vi "Card_output_host.vi"() -> ()   [LabVIEW 2015]
uses:
  <vilib>/userdefined/High Color/nirio_resource_hc.ctl
  <vilib>/FPGAPlugInAG/PXIe-7962R/niLvFpga_Open_PXIe-7962R.vi
  <vilib>/rvi/interface/common/dynamic/niFpgaDynamicAddResources.vi
  <vilib>/LabVIEW Targets/FPGA/FlexRIO/CustomFPGAMethods/79XXR_Method_IOModuleStatusImpl.vi
  <vilib>/Utility/error.llb/Error Cluster From Error Code.vi
  <vilib>/rvi/errors/niLvFpgaAdjustHostInterfaceError.vi
  <vilib>/rvi/interface/common/niFpgaWaitOnOcc.vi
  <instrlib>/_niInstr/Streaming/v1/Host/Public/Start Finite Stream.vi
  <instrlib>/niSync/niSync.llb/niSync Initialize (IVI).vi
  <instrlib>/_niInstr/Streaming/v1/Host/Public/Wait for Stream.vi
  <vilib>/FPGAPlugInAG/Dynamic/niLvFpga_Close_Dynamic.vi
  <vilib>/rvi/interface/nirviOpenFPGA/nirviOpenFPGA.xnode
  FPGA Bitfiles/MochiFPGAControl_FPGATarget_pxie7962fpga_vH47uBXjtQs.lvbitx
  <vilib>/rvi/interface/nirviMethod/nirviMethod.xnode
  <vilib>/rvi/interface/nirviReadWriteControl/nirviReadWriteControl.xnode
  <vilib>/rvi/interface/nirviCloseFPGA/nirviCloseFPGA.xnode
  <instrlib>/_niInstr/Streaming/v1/Host/niInstr Streaming v1 Host.lvlib
  <vilib>/rvi/errors/niLvFpgaMergeErrorWithErrorCode.vi
  <vilib>/rvi/interface/Simulation/niFpgaSimulationCallBeginRW.vi
  NiFpgaLv.dll
  <vilib>/FPGAPlugInAG/Dynamic/niLvFpga_StartFifo_Dynamic.vi
  <vilib>/FPGAPlugInAG/Dynamic/niLvFpga_ReadFifo_Dynamic.vi
  <vilib>/FPGAPlugInAG/Dynamic/niLvFpga_ConfigureFifo_Dynamic.vi
  <vilib>/FPGAPlugInAG/Dynamic/niLvFpga_StopFifo_Dynamic.vi
panel:
  out "subarray":i16[](array[numeric])
  out "size(s) 2":i32[](array[numeric])
  out "size(s)":i32[](array[numeric])
  in  "Trigger destination terminal":string(combo)="PXI_Trig0"
  in  "FPGA":T1 caption="RIO Device"
  out "Bits out DRAM":u64
  out "Writes to DRAM":u64
  in  "?":enum32{"All AI individual", "All AI", "Al 0"}(tab)
  out "AI 31":i32[](graph)
  out "AI 30":i32[](graph)
  out "AI 29":i32[](graph)
  out "AI 28":i32[](graph)
  out "AI 27":i32[](graph)
  out "AI 26":i32[](graph)
  out "AI 25":i32[](graph)
  out "AI 24":i32[](graph)
  out "AI 23":i32[](graph)
  out "AI 22":i32[](graph)
  out "AI 21":i32[](graph)
  out "AI 20":i32[](graph)
  out "AI 19":i32[](graph)
  out "AI 18":i32[](graph)
  out "AI 17":i32[](graph)
  out "AI 16":i32[](graph)
  out "AI 15":i32[](graph)
  out "AI 14":i32[](graph)
  out "AI 13":i32[](graph)
  out "AI 12":i32[](graph)
  out "AI 11":i32[](graph)
  out "AI 10":i32[](graph)
  out "AI 9":i32[](graph)
  out "AI 8":i32[](graph)
  out "AI 7":i32[](graph)
  out "AI 6":i32[](graph)
  out "AI 5":i32[](graph)
  out "AI 4":i32[](graph)
  out "AI 3":i32[](graph)
  out "AI 2":i32[](graph)
  out "AI 1":i32[](graph)
  out "AI 0":i32[](graph)
  out "All AI":waveform(dbl)[](graph)
  out "just AI 1":waveform(dbl)(graph)
  in  "Debug":bool
  out "Bits out DMA":u64
  out "Bits aquired":u64
  out "Writes to DMA":u64
  out "Samples Aquired":u64
  out "Voltage":dbl[][](array[numeric])
  out "Counts":i16[][](array[numeric])
  out "error out":errorcluster
  out "samples transferred":u64
  out "Raw DMA readout":u64[](array[numeric])
  in  "num samples":u64=40000
  in  "Go":bool
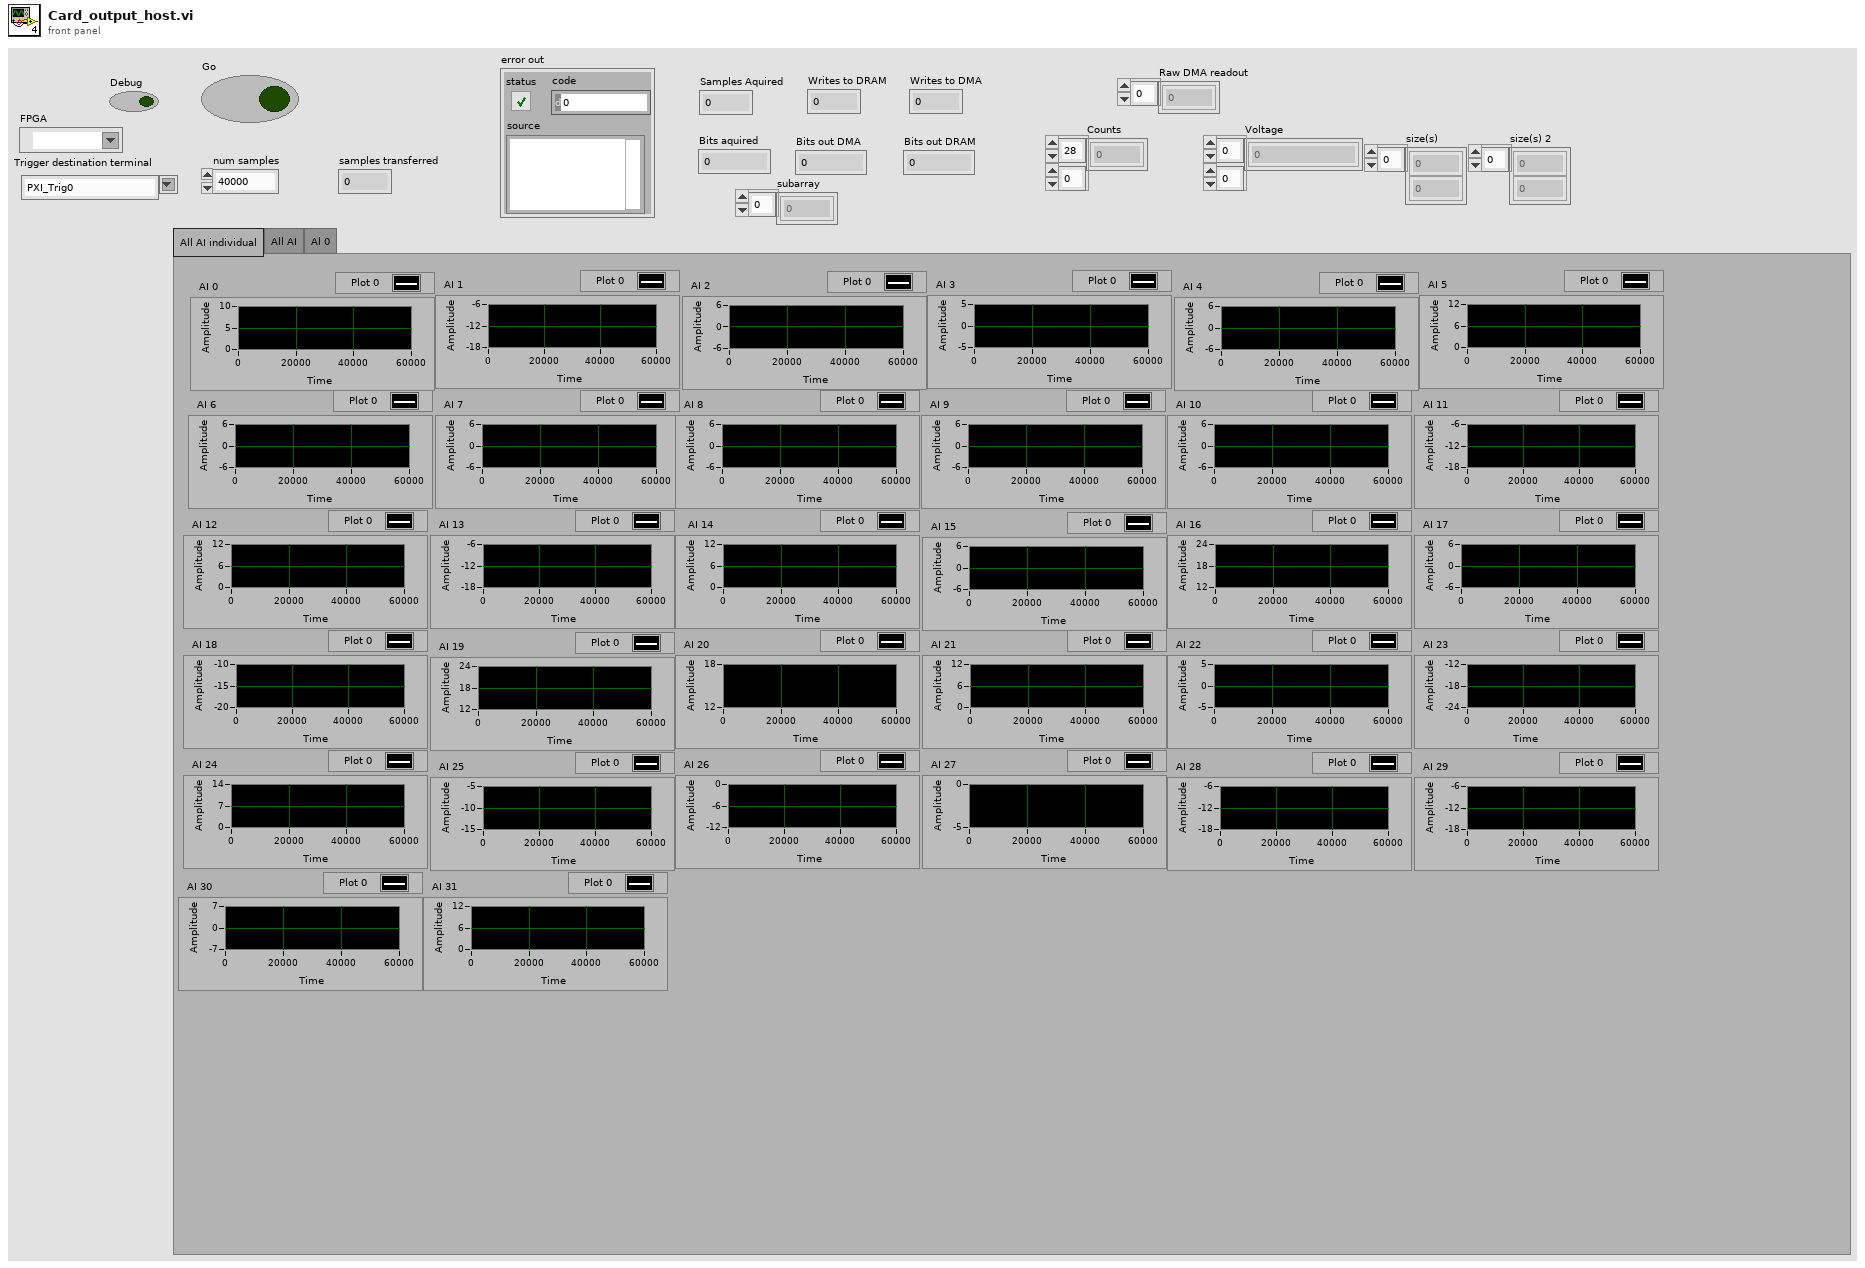
[diagram p1: front panel]
types:
  T1 = typedef "nirio_resource_hc.ctl" = tag
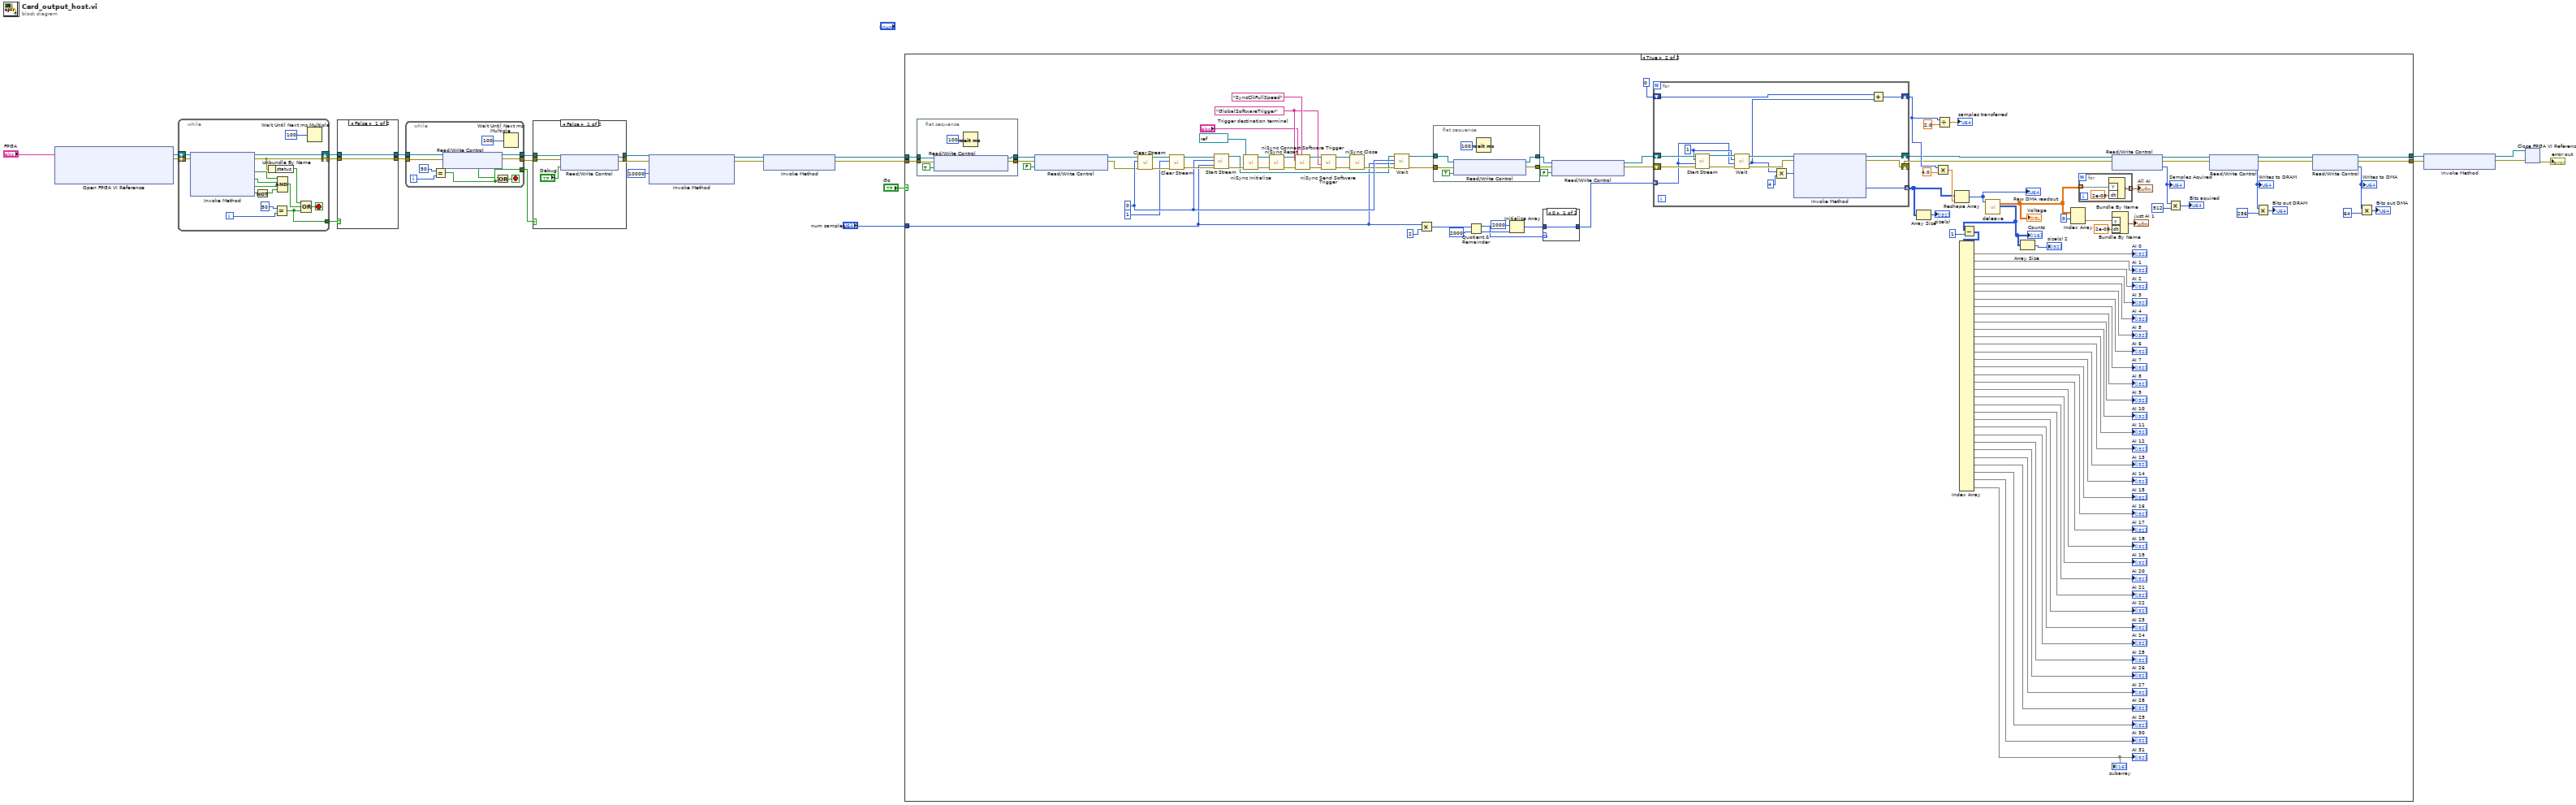
[diagram p0: block diagram]
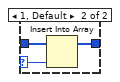
[diagram p3: hidden frame]
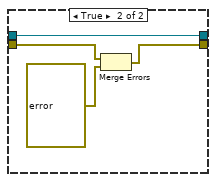
[diagram p4: hidden frame]
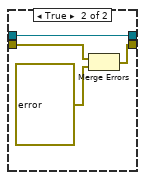
[diagram p5: hidden frame]
diagram:
  n1 = xnode "Open FPGA VI Reference"("resource name"="FPGA") -> ("FPGA VI Reference Out"=w10:refnum<k20>, "error out"=w11:errorcluster)  [unwired: 1 in]
  n2 = while {
    shift-right: [w32] -> w18
    shift-left: w11 -> [w40]
    shift-right: [w39] -> w16
    shift-left: w10 -> [w41]
    tunnel: [w28] -> w17
    i -> [w34]
    stop <- w29 stop-if-true
    n3 = xnode "Invoke Method"("FPGA VI Reference In"=w41, "error in"=w40) -> ("FPGA VI Reference Out"=w39:refnum<k20>, "error out"=w32:errorcluster, "IO Module Present?"=w38:bool, "Power Enabled?"=w37:bool, "IO Enabled?"=w36:bool, "IO Module Mismatch?"=w27:bool)
    n4 = Not(x=w27) -> (.not. x?=w26:bool)
    n5 = Unbundle By Name(w32) -> ("status"=w31:bool)
    n6 = Equal?(x=50, y=w34) -> (x = y?=w28:bool)
    n7 = Compound Arithmetic op=AND(w38, w37, w36, w26) -> (w30:bool)
    n8 = Compound Arithmetic op=OR(w31, w30, w28) -> (w29:bool)
    n9 = Wait Until Next ms Multiple(millisecond multiple=u32 100) -> ()  [unwired: 1 out]
  }
  n10 = case shown="False" w17 {
    tunnel: w18 -> [w42 w46]
    tunnel: [w42 w45] -> w14
    tunnel: w16 -> [w43 w44]
    tunnel: [w43 w44] -> w15
    frame False {
    }
    frame True {
      n11 = Merge Errors(w46, errorcluster {"status"=TRUE, "code"=-1, "source"="The IO Module was not present, powered, or the IO were not enabled.  Verify the NI 5752 is securly connected and try again."} ("error in")) -> (w45:errorcluster)
    }
  }
  n12 = while {
    tunnel: w15 -> [w52]
    tunnel: [w49] -> w8
    tunnel: [w50] -> w7
    tunnel: [w53] -> w9
    tunnel: w14 -> [w51]
    i -> [w56]
    stop <- w54 stop-if-true
    n13 = Equal?(x=50, y=w56) -> (x = y?=w53:bool)
    n14 = xnode "Read/Write Control"("FPGA VI Reference In"=w52, "error in"=w51) -> ("FPGA VI Reference Out"=w49:refnum<k20>, "error out"=w50:errorcluster, "IO Module Init Done"=w48:bool)
    n15 = Or(x=w48, y=w53) -> (x .or. y?=w54:bool)
    n16 = Wait Until Next ms Multiple(millisecond multiple=u32 100) -> ()  [unwired: 1 out]
  }
  n17 = case shown="False" w9 {
    tunnel: w7 -> [w59 w65]
    tunnel: [w58 w64] -> w12
    tunnel: w8 -> [w62 w63]
    tunnel: [w61 w63] -> w13
    frame False {
      n18 = xnode "Read/Write Control"("FPGA VI Reference In"=w62, "error in"=w59, "Output Debug Data"="Debug") -> ("FPGA VI Reference Out"=w61:refnum<k20>, "error out"=w58:errorcluster)
    }
    frame True {
      n19 = Merge Errors(w65, errorcluster {"status"=TRUE, "code"=-1, "source"="The IO Module CLIP was not ready. If you are using any external clocks, make sure they are connected and within the supported specifications."} ("error in")) -> (w64:errorcluster)
    }
  }
  n20 = xnode "Invoke Method"("FPGA VI Reference In"=w13, "error in"=w12, "Requested Depth"=u32 10000) -> ("FPGA VI Reference Out"=w24:refnum<k20>, "error out"=w23:errorcluster)  [unwired: 1 out]
  n21 = xnode "Invoke Method"("FPGA VI Reference In"=w24, "error in"=w23) -> ("FPGA VI Reference Out"=w22:refnum<k20>, "error out"=w21:errorcluster)
  n22 = case shown="True" "Go" {
    tunnel: w22 -> [w68 w161]
    tunnel: "num samples" -> [_ w70]
    tunnel: [w68 w131] -> w4
    tunnel: w21 -> [w67 w130]
    tunnel: [w67 w129] -> w3
    frame False {
      (unwired) errorcluster {"status"=FALSE, "code"=0, "source"=""} ("error out")
    }
    frame True {
      w120 = "GlobalSoftwareTrigger" ("source terminal")
      w176 = 0 ("stream index")
      n23 = flat-sequence {
        tunnel: [w213] -> w164
        tunnel: w161 -> [w212]
        tunnel: [w211] -> w160
        tunnel: w130 -> [w210]
        frame #0 {
          n24 = xnode "Read/Write Control"("FPGA VI Reference In"=w212, "error in"=w210, "Reset DRAM write address"=TRUE) -> ("FPGA VI Reference Out"=w211:refnum<k20>, "error out"=w213:errorcluster)
          n25 = Wait (ms)(milliseconds to wait=u32 100) -> ()  [unwired: 1 out]
        }
      }
      n26 = xnode "Read/Write Control"("FPGA VI Reference In"=w160, "error in"=w164, "Reset DRAM write address"=FALSE) -> ("FPGA VI Reference Out"=w140:refnum<k20>, "error out"=w145:errorcluster)
      n27 = call <instrlib>:"Clear Stream.vi"("error in (no error)"=w145, "stream index"=w176, "refnum in"=w140) -> ("error out"=w179:errorcluster, "refnum out"=w180:refnum<k20>)  [unwired: 7 in]
      n28 = call <instrlib>:"Clear Stream.vi"("error in (no error)"=w179, "stream index"=1, "refnum in"=w180) -> ("error out"=w177:errorcluster, "refnum out"=w178:refnum<k20>)  [unwired: 7 in]
      n29 = call-poly <instrlib>:"Start Stream.vi"("error in (no error)"=w177, "num samples"=w70, "stream index"=w176, "refnum in"=w178) -> ("error out"=w126:errorcluster, "refnum out"=w119:refnum<k20>)  [unwired: 6 in]
      n30 = call-poly <instrlib>:"niSync Initialize.vi"("error in (no error)"=w126, "resource name"=refnum<k15> "Sync1") -> ("error out"=w77:errorcluster, "instrument handle out"=w78:refnum<k15>)  [unwired: 8 in]
      n31 = call <instrlib>:"niSync Reset.vi"("error in (no error)"=w77, "instrument handle"=w78) -> ("error out"=w75:errorcluster, "instrument handle out"=w76:refnum<k15>)  [unwired: 8 in]
      n32 = call <instrlib>:"niSync Connect Software Trigger.vi"("synchronization clock"="SyncClkFullSpeed", "error in (no error)"=w75, "destination terminal"="Trigger destination terminal", "source terminal"=w120, "instrument handle"=w76) -> ("error out"=w128:errorcluster, "instrument handle out"=w127:refnum<k15>)  [unwired: 5 in]
      n33 = call <instrlib>:"niSync Send Software Trigger.vi"("error in (no error)"=w128, "source terminal"=w120, "instrument handle"=w127) -> ("error out"=w124:errorcluster, "instrument handle out"=w125:refnum<k15>)  [unwired: 7 in]
      n34 = call <instrlib>:"niSync Close.vi"("error in (no error)"=w124, "instrument handle"=w125) -> ("error out"=w123:errorcluster)  [unwired: 9 in]
      n35 = call-poly <instrlib>:"Wait.vi"("error in (no error)"=w123, "wait for samples transferred"=w70, "stream index"=w176, "refnum in"=w119) -> ("error out"=w69:errorcluster, "refnum out"=w159:refnum<k20>)  [unwired: 4 in, 2 out]
      n36 = Multiply(x=w70, y=u64 2) -> (x*y=w151:u64)
      n37 = flat-sequence {
        tunnel: [w207] -> w162
        tunnel: w159 -> [w206]
        tunnel: [w205] -> w158
        tunnel: w69 -> [w204]
        frame #0 {
          n38 = xnode "Read/Write Control"("FPGA VI Reference In"=w206, "error in"=w204, "Reset DRAM read address"=TRUE ("Reset DRAM write address")) -> ("FPGA VI Reference Out"=w205:refnum<k20>, "error out"=w207:errorcluster)
          n39 = Wait (ms)(milliseconds to wait=u32 100) -> ()  [unwired: 1 out]
        }
      }
      n40 = Quotient & Remainder(x=w151, y=u64 2000) -> (x-y*floor(x/y)=w141:u64, floor(x/y)=w149:u64)
      n41 = Initialize Array(u64 2000 ("element"), w149) -> (w147:u64[])
      n42 = case shown="0" w141 {
        selector: w141 -> [_ w185]
        tunnel: w147 -> [w184 w187]
        tunnel: [w184 w186] -> w146
        frame 0 {
        }
        frame 1, Default {
          n43 = Insert Into Array(array=w187, new element=w185) -> (w186:u64[])  [unwired: 1 in]
        }
      }
      n44 = xnode "Read/Write Control"("FPGA VI Reference In"=w158, "error in"=w162, "Reset DRAM read address"=FALSE ("Reset DRAM write address")) -> ("FPGA VI Reference Out"=w152:refnum<k20>, "error out"=w153:errorcluster)
      n45 = for {
        shift-right: [w190] -> w144
        shift-left: w152 -> [w200]
        shift-right: [w189] -> w139
        shift-left: w153 -> [w199]
        shift-right: [w203] -> w155
        shift-left: u64 0 -> [w197]
        tunnel: w146 -> [w188] mode=indexing
        tunnel: [w191] -> w81 mode=indexing
        w198 = 1 ("stream index")
        n46 = call-poly <instrlib>:"Start Stream.vi"("error in (no error)"=w199, "num samples"=w188, "stream index"=w198, "refnum in"=w200) -> ("error out"=w201:errorcluster, "refnum out"=w202:refnum<k20>)  [unwired: 6 in]
        n47 = call-poly <instrlib>:"Wait.vi"("error in (no error)"=w201, "wait for samples transferred"=w188, "stream index"=w198, "refnum in"=w202) -> ("error out"=w195:errorcluster, "samples transferred"=w193:u64, "refnum out"=w196:refnum<k20>)  [unwired: 4 in, 1 out]
        n48 = Multiply(x=w193, y=u64 4) -> (x*y=w194:u64)
        n49 = xnode "Invoke Method"("FPGA VI Reference In"=w196, "error in"=w195, "Number of Elements"=w194) -> ("FPGA VI Reference Out"=w190:refnum<k20>, "error out"=w189:errorcluster, "Data"=w191:u64[])  [unwired: 1 in, 1 out]
        n50 = Add(x=w197, y=w193) -> (x+y=w203:u64)
      }
      n51 = Array Size(array=w81) -> (size(s)=→"size(s)":i32[])
      n52 = Multiply(x=w155, y=4.0) -> (x*y=w143:dbl)
      n53 = Divide(x=w155, y=2.0) -> (x/y=→"samples transferred":dbl)
      n54 = Reshape Array(w81, w143) -> (w142:u64[])
      "Raw DMA readout" <- w142
      n55 = call "deleave.vi"("Data"=w142) -> ("Counts"=w73:i16[][], "Voltage"=w74:dbl[][])  [unwired: 9 in]
      "Voltage" <- w74
      "Counts" <- w73
      n56 = Subtract(x=w73, y=1) -> (x-y=w71:i32[][])
      n57 = Index Array(array=w71) -> (element #1=→"AI 0":i32[], element #2=→"AI 1":i32[], element #3=→"AI 2":i32[], element #4=→"AI 3":i32[], element #5=→"AI 4":i32[], element #6=→"AI 5":i32[], element #7=→"AI 6":i32[], element #8=→"AI 7":i32[], element #9=→"AI 8":i32[], element #10=→"AI 9":i32[], element #11=→"AI 10":i32[], element #12=→"AI 11":i32[], element #13=→"AI 12":i32[], element #14=→"AI 13":i32[], element #15=→"AI 14":i32[], element #16=→"AI 15":i32[], element #17=→"AI 16":i32[], element #18=→"AI 17":i32[], element #19=→"AI 18":i32[], element #20=→"AI 19":i32[], element #21=→"AI 20":i32[], element #22=→"AI 21":i32[], element #23=→"AI 22":i32[], element #24=→"AI 23":i32[], element #25=→"AI 24":i32[], element #26=→"AI 25":i32[], element #27=→"AI 26":i32[], element #28=→"AI 27":i32[], element #29=→"AI 28":i32[], element #30=→"AI 29":i32[], element #31=→"AI 30":i32[], element #32=→"AI 31" →"subarray":i32[])  [unwired: 64 in]
      n58 = Array Size(array=w73) -> (size(s)=→"size(s) 2":i32[])
      n59 = Index Array(array=w74, index (row)=0) -> (element=w117:dbl[])  [unwired: 1 in]
      n60 = for {
        tunnel: [w183] -> w115 mode=indexing
        tunnel: w74 -> [w182] mode=indexing
        n61 = Bundle By Name("Y"=w182, "dt"=2e-08) -> (w183:waveform(dbl))  [unwired: 1 in]
      }
      "All AI" <- w115
      n62 = xnode "Read/Write Control"("FPGA VI Reference In"=w144, "error in"=w139) -> ("FPGA VI Reference Out"=w135:refnum<k20>, "error out"=w134:errorcluster, "Samples Aquired"=w172:u64)
      "Samples Aquired" <- w172
      n63 = Bundle By Name("Y"=w117, "dt"=2e-08) -> (→"just AI 1":waveform(dbl))  [unwired: 1 in]
      n64 = Multiply(x=w172, y=u64 512) -> (x*y=→"Bits aquired":u64)
      n65 = xnode "Read/Write Control"("FPGA VI Reference In"=w135, "error in"=w134) -> ("FPGA VI Reference Out"=w133:refnum<k20>, "error out"=w132:errorcluster, "Writes to DRAM"=w137:u64)
      "Writes to DRAM" <- w137
      n66 = Multiply(x=w137, y=u64 256) -> (x*y=→"Bits out DRAM":u64)
      n67 = xnode "Read/Write Control"("FPGA VI Reference In"=w133, "error in"=w132) -> ("FPGA VI Reference Out"=w131:refnum<k20>, "error out"=w129:errorcluster, "Writes to DMA"=w169:u64)
      "Writes to DMA" <- w169
      n68 = Multiply(x=w169, y=u64 64) -> (x*y=→"Bits out DMA":u64)
    }
  }
  n69 = xnode "Invoke Method"("FPGA VI Reference In"=w4, "error in"=w3) -> ("FPGA VI Reference Out"=w1:refnum<k20>, "error out"=w2:errorcluster)
  n70 = xnode "Close FPGA VI Reference"("FPGA VI Reference In"=w1, "error in"=w2) -> ("error out"=→"error out":errorcluster)
